vi "API - Check Packet ID Conflict.vi"(7 "Transmit?":bool, 8 "error in (no error)":errorcluster, 10 "New ID":i32, 11 "Packet Ref In":T1=18446744073709551615 format="%.0x") -> (0 "error out":errorcluster, 2 "Conflicting ID?":bool)   [LabVIEW 2016, in "UDP-Custom-Device System Explorer.lvlib"]
uses:
  UDP-Custom-Device System Explorer.lvlib
  <vilib>/NI Veristand/Custom Device API/Custom Device Item Ref.ctl
  Shared/Constants.vi
  <vilib>/NI Veristand/Custom Device API/Get Item Property (I32).vi
  <vilib>/NI VeriStand/Custom Device API/Custom Device API.lvlib
  Shared/UDP-Custom-Device Shared.lvlib
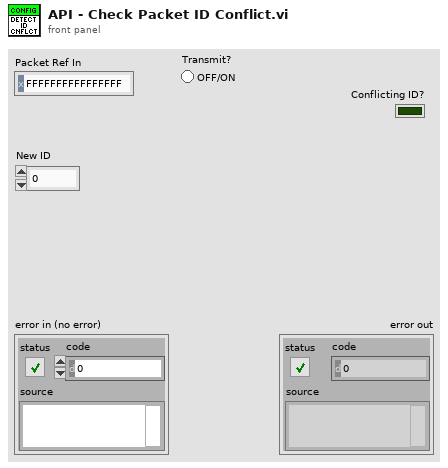
[diagram p1: front panel]
types:
  T1 = typedef "Custom Device API.lvlib/Custom Device Item Ref.ctl" = u64
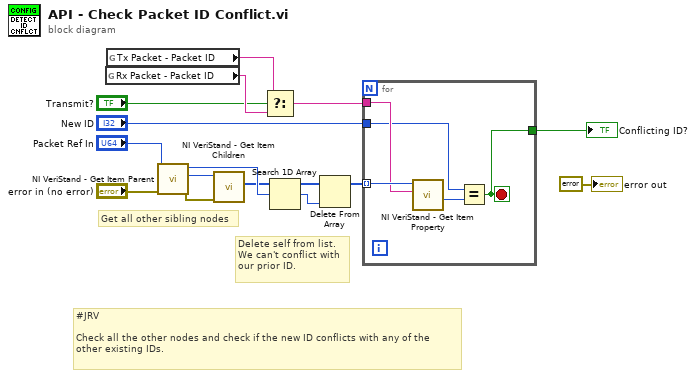
[diagram p0: block diagram]
diagram:
  # "Delete self from list.\nWe can't conflict with\nour prior ID."
  # "Get all other sibling nodes"
  # "#JRV\n\nCheck all the other nodes and check if the new ID conflicts with any of the\nother existing IDs."
  n1 = global read "Constants.vi" "Rx Packet - Packet ID"() -> (w5:string)
  n2 = global read "Constants.vi" "Tx Packet - Packet ID"() -> (w6:string)
  n3 = call <vilib>:"NI VeriStand - Get Item Parent.vi"("error in (no error)"="error in (no error)", "Item Ref in"="Packet Ref In") -> ("error out"=w12:errorcluster, "Parent Ref"=w13:T1, "Item Ref out"=w11:T1)  [unwired: 6 in, 1 out]
  n4 = call <vilib>:"NI VeriStand - Get Item Children.vi"("error in (no error)"=w12, "Item Ref in"=w13) -> ("Child Refs"=w10:T1[])  [unwired: 6 in, 3 out]
  n5 = Select(t=w6, s="Transmit?", f=w5) -> (s? t:f=w3:string)
  n6 = Search 1D Array(1D array=w10, element=w11) -> (index of element=w9:i32)  [unwired: 1 in]
  n7 = Delete From Array(array=w10, index=w9) -> (array with subset deleted=w8:T1[])  [unwired: 1 in, 1 out]
  n8 = for {
    tunnel: w8 -> [w20] mode=indexing
    tunnel: "New ID" -> [w17]
    tunnel: w3 -> [w19]
    tunnel: [w16] -> w2
    stop <- w16 stop-if-true
    n9 = call-poly <vilib>:"NI VeriStand - Get Item Property.vi"("Property Name"=w19, "Item Ref in"=w20) -> ("Value"=w18:i32)  [unwired: 6 in, 3 out]
    n10 = Equal?(x=w17, y=w18) -> (x = y?=w16:bool)
  }
  "Conflicting ID?" <- w2
  "error out" <- errorcluster {"status"=FALSE, "code"=0, "source"=""} ("error out")
